vi "InitSelfCheck.vi"() -> ()   [LabVIEW 2014]
uses:
  <vilib>/addons/database/Connection.llb/DB Tools Open Connec (String).vi
  <vilib>/addons/database/Connection.llb/Conn Execute.vi
  <vilib>/addons/database/Recordset.llb/Rec Fetch Recordset Data (R).vi
  <vilib>/addons/database/Recordset.llb/Rec Destroy - Connection.vi
  <vilib>/addons/database/_DB Variant To Data/Database Variant To Data.xnode
  <vilib>/Instr/_visa.llb/VISA Configure Serial Port (Instr).vi
  <vilib>/addons/database/NI_Database_API.lvlib
panel:
  out "错误输出 2":errorcluster caption="错误输出"
  out "String":string
  out "Slide":u8(slide) scale=0.0..50.0
  out "Current Status":string
  # "自检中...请稍候\n\n\n--"
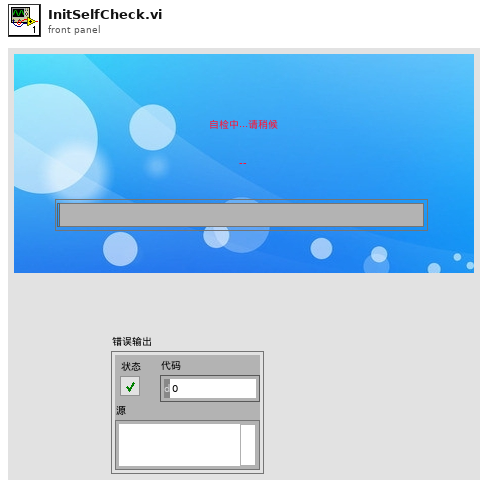
[diagram p1: front panel]
types:
  T1 = typedef "NI_Database_API.lvlib/Conn ObjectReference.ctl" = refnum<k1>
  T2 = typedef "NI_Database_API.lvlib/Rec ObjectReference.ctl" = refnum<k1>
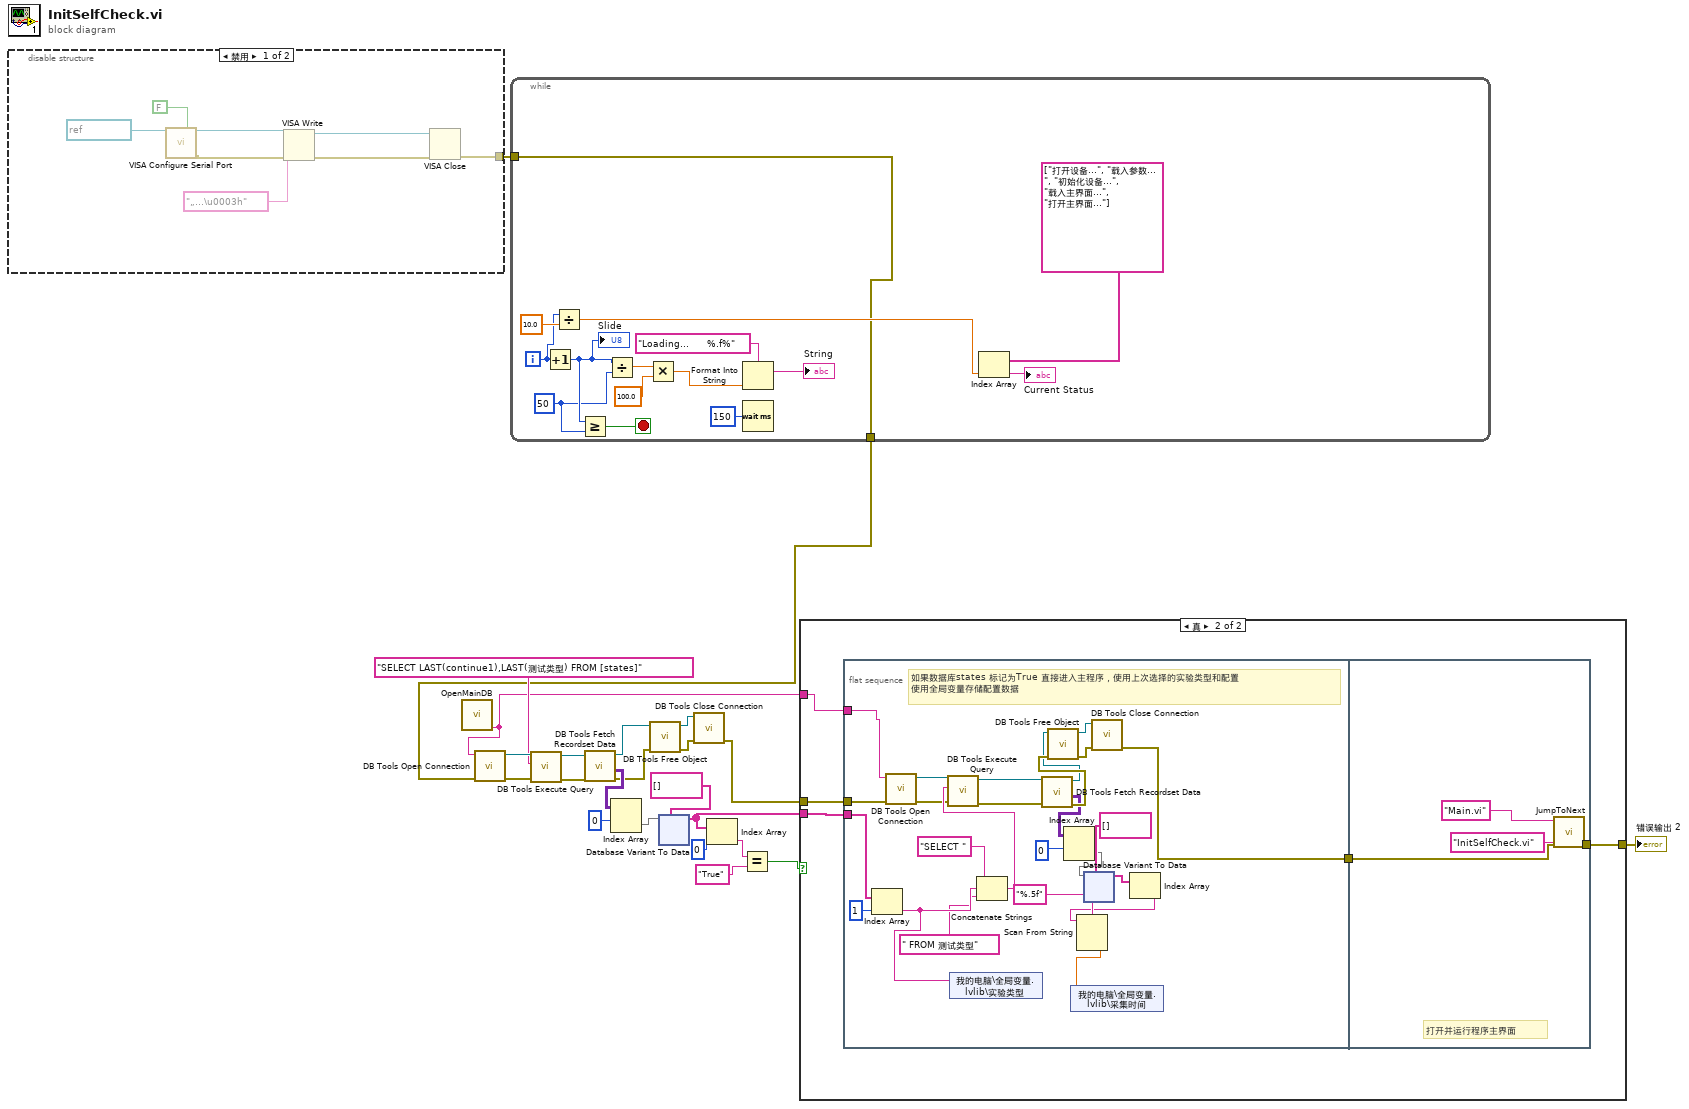
[diagram p0: block diagram]
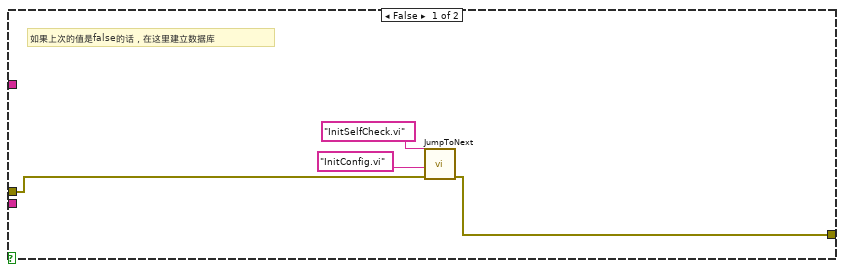
[diagram p3: hidden frame]
diagram:
  n1 = disable-structure shown="禁用" {
    disable-tunnel: [w24 _] -> w1
    frame Disabled {
      n2 = call-poly "VISA Configure Serial Port"("VISA resource name"=refnum<visa-resource-name> "COM2", "Enable Termination\nChar (T)"=FALSE ("Enable Termination\nChar (T)")) -> ("VISA resource name out"=w29:refnum<visa-resource-name>, "error out"=w28:errorcluster)  [unwired: 12 in]
      n3 = VISA Write(VISA resource name=w29, write buffer="„…\u0003h" ("写入缓冲区"), error in (no error)=w28) -> (VISA resource name out=w30:refnum<visa-resource-name>, error out=w31:errorcluster)  [unwired: 1 out]
      n4 = VISA Close(VISA resource name=w30, error in (no error)=w31) -> (error out=w24:errorcluster)
    }
    frame Enabled {
    }
  }
  n5 = call "OpenMainDB.vi"() -> ("头信息"=w5:string)  [unwired: 11 in]
  n6 = while {
    tunnel: [w32] -> w2
    tunnel: w1 -> [w32]
    i -> [w34]
    stop <- w44 stop-if-true
    w41 = 50 ("y")
    n7 = Increment(x=w34) -> (x+1=w43:i32)
    "Slide" <- w43
    n8 = Divide(x=w34, y=10.0) -> (x/y=w33:dbl)
    n9 = Greater Or Equal?(x=w43, y=w41) -> (x >= y?=w44:bool)
    n10 = Divide(x=w43, y=w41) -> (x/y=w42:dbl)
    n11 = Multiply(x=w42, y=100.0) -> (x*y=w39:dbl)
    n12 = Format Into String(format string="Loading...      %.f%", w39) -> (resulting string=→"String":string)  [unwired: 2 in, 1 out]
    n13 = Wait (ms)(milliseconds to wait=u32 150) -> ()  [unwired: 1 out]
    n14 = Index Array(array=string[] ["打开设备...", "载入参数...", "初始化设备...", "载入主界面...", "打开主界面..."], index=w33) -> (element=→"Current Status":string)
  }
  n15 = call-poly <vilib>:"DB Tools Open Connection.vi"("error in (no error)"=w2, "connection information"=w5) -> ("error out"=w23:errorcluster, "connection reference"=w22:T1)  [unwired: 6 in]
  n16 = call-poly <vilib>:"DB Tools Execute Query.vi"("error in (no error)"=w23, "SQL query"="SELECT LAST(continue1),LAST(测试类型) FROM [states]", "connection reference"=w22) -> ("error out"=w19:errorcluster, "recordset reference"=w20:T2)  [unwired: 5 in]
  n17 = call-poly <vilib>:"DB Tools Fetch Recordset Data.vi"("error in (no error)"=w19, "recordset reference"=w20) -> ("error out"=w9:errorcluster, "recordset data"=w18:variant[][], "recordset reference out"=w10:T2)  [unwired: 3 in]
  n18 = Index Array(array=w18, index (row)=0 ("索引 (行)")) -> (element=w16:variant[])  [unwired: 1 in]
  n19 = call-poly <vilib>:"DB Tools Free Object.vi"("error in (no error)"=w9, "recordset reference"=w10) -> ("error out"=w7:errorcluster, "connection reference"=w8:T1)  [unwired: 8 in]
  n20 = xnode "Database Variant To Data"("database variant"=w16, "type"=string[] []) -> ("data"=w6:string[])  [unwired: 1 in, 1 out]
  n21 = call <vilib>:"DB Tools Close Connection.vi"("error in (no error)"=w7, "connection reference"=w8) -> ("error out"=w4:errorcluster)  [unwired: 5 in]
  n22 = Index Array(array=w6, index=0 ("索引")) -> (element=w13:string)
  n23 = Equal?(x=w13, y="True") -> (x = y?=w11:bool)
  n24 = case shown="真" w11 {
    tunnel: w6 -> [_ w54]
    tunnel: w5 -> [_ w55]
    tunnel: w4 -> [w48 w53]
    tunnel: [w47 w51] -> w3
    frame False {
      # "如果上次的值是false的话，在这里建立数据库"
      n25 = call "JumpToNext.vi"("错误输入（无错误）"=w48, "要关闭的VI"="InitSelfCheck.vi", "要打开的VI"="InitConfig.vi") -> ("错误输出"=w47:errorcluster)  [unwired: 8 in]
    }
    frame True {
      n26 = flat-sequence {
        tunnel: w55 -> [w59]
        tunnel: w54 -> [w58]
        tunnel: w53 -> [w57]
        tunnel: [w56] -> w52
        tunnel: w52 -> [w120]
        tunnel: [w119] -> w51
        frame #0 {
          # "如果数据库states 标记为True 直接进入主程序，使用上次选择的实验类型和配置\n使用全局变量存储配置数据"
          n27 = Index Array(array=w58, index=1 ("索引")) -> (element=w80:string)
          n28 = call-poly <vilib>:"DB Tools Open Connection.vi"("error in (no error)"=w57, "connection information"=w59) -> ("error out"=w62:errorcluster, "connection reference"=w61:T1)  [unwired: 6 in]
          n29 = shared-variable "我的电脑\\全局变量.lvlib\\实验类型"(w80) -> ()  [unwired: 1 in, 1 out]
          n30 = Concatenate Strings("SELECT ", w80, " FROM 测试类型") -> (w65:string)
          n31 = call-poly <vilib>:"DB Tools Execute Query.vi"("error in (no error)"=w62, "SQL query"=w65, "connection reference"=w61) -> ("error out"=w67:errorcluster, "recordset reference"=w66:T2)  [unwired: 5 in]
          n32 = call-poly <vilib>:"DB Tools Fetch Recordset Data.vi"("error in (no error)"=w67, "recordset reference"=w66) -> ("error out"=w76:errorcluster, "recordset data"=w69:variant[][], "recordset reference out"=w75:T2)  [unwired: 3 in]
          n33 = call-poly <vilib>:"DB Tools Free Object.vi"("error in (no error)"=w76, "recordset reference"=w75) -> ("error out"=w73:errorcluster, "connection reference"=w74:T1)  [unwired: 8 in]
          n34 = Index Array(array=w69, index (row)=0 ("索引 (行)")) -> (element=w70:variant[])  [unwired: 1 in]
          n35 = xnode "Database Variant To Data"("database variant"=w70, "type"=string[] []) -> ("data"=w72:string[])  [unwired: 1 in, 1 out]
          n36 = call <vilib>:"DB Tools Close Connection.vi"("error in (no error)"=w73, "connection reference"=w74) -> ("error out"=w56:errorcluster)  [unwired: 5 in]
          n37 = Index Array(array=w72) -> (element=w77:string)  [unwired: 1 in]
          n38 = Scan From String(format string="%.5f" ("格式字符串"), input string=w77) -> (output 1=w79:dbl)  [unwired: 3 in, 3 out]
          n39 = shared-variable "我的电脑\\全局变量.lvlib\\采集时间"(w79) -> ()  [unwired: 1 in, 1 out]
        }
        frame #1 {
          # "打开并运行程序主界面"
          n40 = call "JumpToNext.vi"("错误输入（无错误）"=w120, "要关闭的VI"="InitSelfCheck.vi", "要打开的VI"="Main.vi") -> ("错误输出"=w119:errorcluster)  [unwired: 8 in]
        }
      }
    }
  }
  "错误输出 2" <- w3
